vi "Start Move.vi"(8 "error in (no error)":errorcluster, 11 "ScrollingList in":refnum<class "ScrollingList.lvclass">) -> (0 "error out":errorcluster, 2 "Button Down":bool, 3 "ScrollingList (dup)":refnum<class "ScrollingList.lvclass">)   [LabVIEW 2020, in "ScrollingList.lvclass"]
uses:
  ScrollingList.lvclass
  ScrollingList.lvclass/ScrollingList.ctl
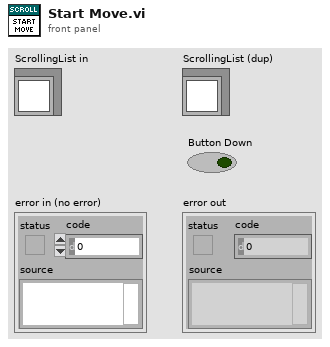
[diagram p1: front panel]
types:
  T1 = typedef "LVMouseTypeDef.ctl" = cluster{"Mouse Position":cluster{"X":i32, "Y":i32}, "Mouse Modifiers":cluster{"Button Down":bool, "Shift Mod":bool, "Menu Mod":bool, "Option Mod":bool}}
  T2 = typedef "ScrollingList.lvclass/State Data.ctl" = cluster{"Timeout":i32, "Time":timestamp, "Y":i32, "Origin:Top":i16, "Rate":dbl, "ListItems":string[], "Item Height":i32, "Max Height":i32}
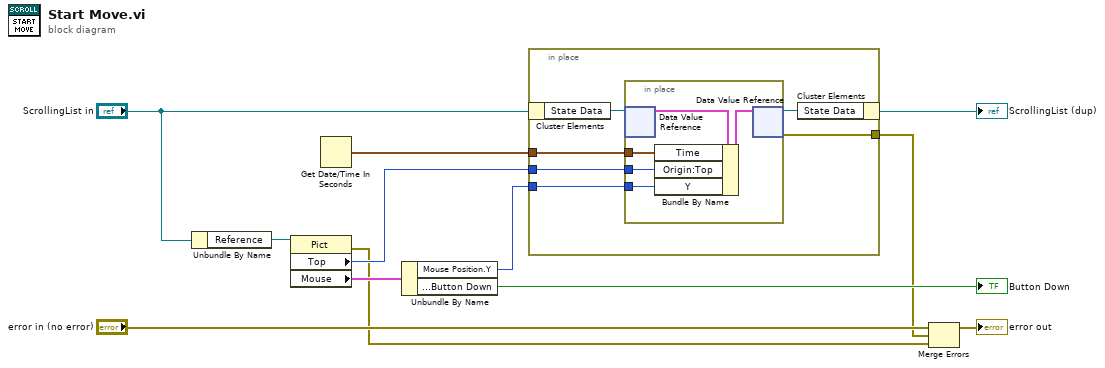
[diagram p0: block diagram]
diagram:
  n1 = Unbundle By Name("ScrollingList in") -> ("Reference"=w10:refnum<vi>)
  n2 = property on="Property Node" class="Pict"(reference=w10) -> (error out=w1:errorcluster, "Top"=w4:i16, "Mouse"=w9:T1)  [unwired: 1 in, 1 out]
  n3 = Get Date/Time In Seconds() -> (seconds since 1Jan1904=w6:timestamp)
  n4 = Unbundle By Name(w9) -> ("Mouse Position.Y"=w5:i32, "Mouse Modifiers.Button Down"=→"Button Down":bool)
  n5 = in-place {
    in-place-border: w6 -> [w16]
    in-place-border: w5 -> [w15]
    in-place-border: w4 -> [w14]
    in-place-border: [w13] -> w2
    n6 = in-place-cluster #1("ScrollingList in") -> ("State Data"=w18:refnum<data-value>)
    n7 = in-place {
      in-place-border: w16 -> [w21]
      in-place-border: w15 -> [w20]
      in-place-border: w14 -> [w19]
      n8 = in-place-dvr #2(w18) -> (w23:T2)  [unwired: 1 out]
      n9 = Bundle By Name(cluster=w23, "Time"=w21, "Origin:Top"=w19, "Y"=w20) -> (w22:T2)
      n10 = in-place-dvr #2(w22) -> (w17:refnum<data-value>, w13:errorcluster)
    }
    n11 = in-place-cluster #1("State Data"=w17) -> (→"ScrollingList (dup)":refnum<class "ScrollingList.lvclass">)
  }
  n12 = Merge Errors("error in (no error)", w2, w1) -> (→"error out":errorcluster)
